vi "Disconnect Targets.vi"(8 "error in":errorcluster, 10 "Disconnect targets":string[](array[string]), 11 "2525 in":refnum<class "2525.lvclass">) -> (0 "error out":errorcluster, 3 "2525 out":refnum<class "2525.lvclass">)   [LabVIEW 2019, in "2525.lvlib" / "2525.lvclass"]
uses:
  Library/2525.lvclass
  Library/2525.lvclass/2525.ctl
  <instrlib>/niSwitch/niSwitch.llb/niSwitch Disconnect Channels (Single).vi
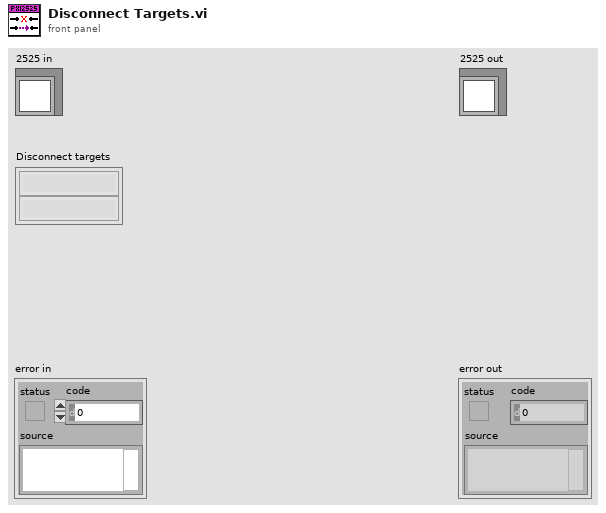
[diagram p1: front panel]
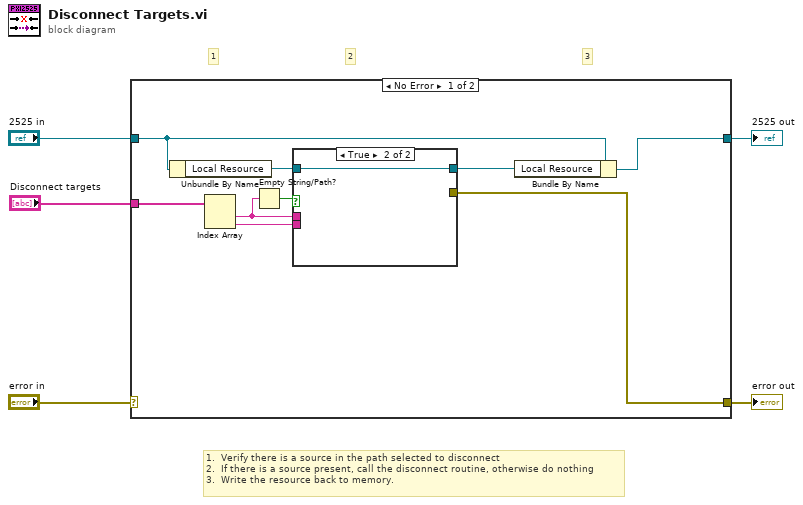
[diagram p0: block diagram]
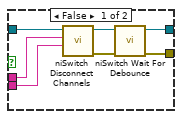
[diagram p2: hidden frame]
diagram:
  # "1.  Verify there is a source in the path selected to disconnect\n2.  If there is a source present, call the disconnect routine, otherwise do nothing\n3.  Write the resource back to memory."
  # "3"
  # "2"
  # "1"
  n1 = case shown="No Error" "error in" {
    selector: "error in" -> [_ w24]
    tunnel: [w8 w24] -> w4
    tunnel: [w10 w23] -> w2
    tunnel: "2525 in" -> [w13 w23]
    tunnel: "Disconnect targets" -> [w14 _]
    frame No Error {
      n2 = Unbundle By Name(w13) -> ("Local Resource"=w12:refnum<k15>)
      n3 = Index Array(array=w14) -> (element #1=w6:string, element #2=w11:string)  [unwired: 2 in]
      n4 = Empty String/Path?(string/path=w6) -> (empty?=w7:bool)
      n5 = case shown="True" w7 {
        tunnel: w12 -> [w21 w22]
        tunnel: w6 -> [w18 _]
        tunnel: w11 -> [w17 _]
        tunnel: [w16 w22] -> w9
        tunnel: [w15 _] -> w8
        frame False {
          n6 = call-poly <instrlib>:"niSwitch Disconnect Channels.vi"("channel 2"=w17, "channel 1"=w18, "instrument handle"=w21) -> ("error out"=w20:errorcluster, "instrument handle out"=w19:refnum<k15>)  [unwired: 7 in]
          n7 = call <instrlib>:"niSwitch Wait For Debounce.vi"("error in (no error)"=w20, "instrument handle"=w19) -> ("error out"=w15:errorcluster, "instrument handle out"=w16:refnum<k15>)  [unwired: 8 in]
        }
        frame True {
        }
      }
      n8 = Bundle By Name(cluster=w13, "Local Resource"=w9) -> (w10:refnum<class "2525.lvclass">)
    }
    frame Error {
    }
  }
  "error out" <- w4
  "2525 out" <- w2
